vi "IO@SetPort__Parameter.vi"(1 "ParamterIn":string) -> (0 "ParamterOut":string)   [LabVIEW 2020]
panel:
  in  "ForceUpdate":string(combo)
  in  "Delay":string(combo)
  in  "PortSelect":string(combo)
  in  "Confirm":bool
  # "IO@SetPort/ClrPort $IOName(,$Delay,ForceUpdate)"
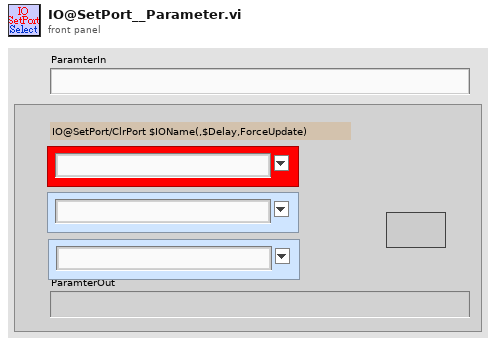
[diagram p1: front panel]
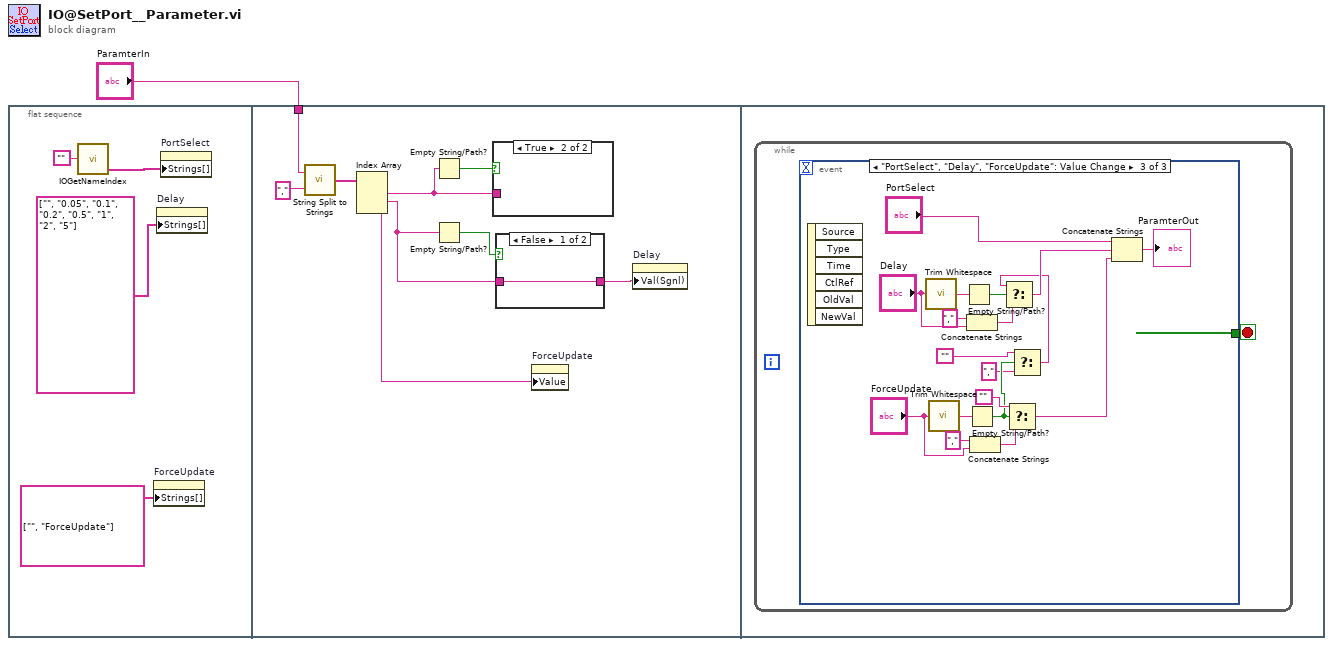
[diagram p0: block diagram]
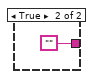
[diagram p2: hidden frame]
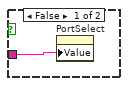
[diagram p3: hidden frame]
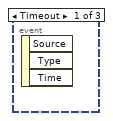
[diagram p4: hidden frame]
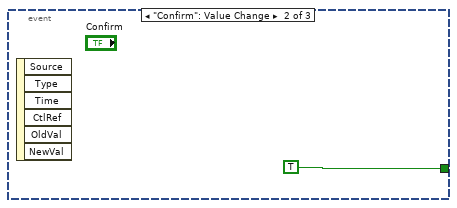
[diagram p5: hidden frame]
diagram:
  n1 = flat-sequence {
    tunnel: "ParamterIn" -> [w12]
    frame #0 {
      n2 = call "IOGetNameIndex.vi"("PortName"="") -> ("PortNameList Out"=w4:string[])  [unwired: 3 in, 1 out]
      n3 = property on="ForceUpdate" class="CmbBox"("Strings[]"=string[] ["", "ForceUpdate"] ("Strings []")) -> ()  [unwired: 2 in, 2 out]
      n4 = property on="Delay" class="CmbBox"("Strings[]"=string[] ["", "0.05", "0.1", "0.2", "0.5", "1", "2", "5"] ("Strings []")) -> ()  [unwired: 2 in, 2 out]
      n5 = property on="PortSelect" class="CmbBox"("Strings[]"=w4) -> ()  [unwired: 2 in, 2 out]
    }
    frame #1 {
      n6 = call "String Split to Strings.vi"("search string/char (-)"=",", "String"=w12) -> ("Array"=w13:string[])
      n7 = Index Array(array=w13) -> (element #1=w10:string, element #2=w7:string, element #3=w6:string)  [unwired: 3 in]
      n8 = Empty String/Path?(string/path=w10) -> (empty?=w11:bool)
      n9 = Empty String/Path?(string/path=w7) -> (empty?=w9:bool)
      n10 = case shown="True" w11 {
        tunnel: w10 -> [w17 _]
        frame False {
          n11 = property on="PortSelect" class="CmbBox"("Value"=w17) -> ()  [unwired: 2 in, 2 out]
        }
        frame True {
        }
      }
      n12 = case shown="False" w9 {
        tunnel: [w15 ""] -> w8
        tunnel: w7 -> [w15 _]
        frame False {
        }
        frame True {
        }
      }
      n13 = property on="ForceUpdate" class="CmbBox"("Value"=w6) -> ()  [unwired: 2 in, 2 out]
      n14 = property on="Delay" class="CmbBox"("Val(Sgnl)"=w8) -> ()  [unwired: 2 in, 2 out]
    }
    frame #2 {
      n15 = while {
        stop <- w18 stop-if-true
        n16 = event shown="[2] \"PortSelect\", \"Delay\", \"ForceUpdate\": Value Change" {
          selector: _ -> [_ _ _]
          dyn-events: _ -> [_ _ _]
          timeout: _ -> [_ _ _]
          tunnel: [_ TRUE _] -> w18
          event Timeout {
            n17 = event-data() -> ()  [unwired: 1 in, 3 out]
          }
          event "Confirm": Value Change {
            n18 = event-data() -> ()  [unwired: 1 in, 6 out]
          }
          event "PortSelect", "Delay", "ForceUpdate": Value Change {
            n19 = event-data() -> ()  [unwired: 1 in, 6 out]
            n20 = call <vilib>:"Trim Whitespace.vi"("string"="Delay") -> ("trimmed string"=w35:string)  [unwired: 1 in]
            n21 = call <vilib>:"Trim Whitespace.vi"("string"="ForceUpdate") -> ("trimmed string"=w27:string)  [unwired: 1 in]
            n22 = Empty String/Path?(string/path=w35) -> (empty?=w34:bool)
            n23 = Concatenate Strings("," ("string"), "Delay") -> (w33:string)
            n24 = Empty String/Path?(string/path=w27) -> (empty?=w24:bool)
            n25 = Concatenate Strings("," ("string"), "ForceUpdate") -> (w29:string)
            n26 = Select(t="", s=w24, f=w29) -> (s? t:f=w20:string)
            n27 = Select(t="", s=w24, f=",") -> (s? t:f=w21:string)
            n28 = Select(t=w21, s=w34, f=w33) -> (s? t:f=w25:string)
            n29 = Concatenate Strings("PortSelect", w25, w20) -> (→"ParamterOut":string)
          }
        }
      }
    }
  }
